vi "Scan DQMH Modules.vi"(8 "error in":errorcluster) -> (0 "error out":errorcluster, 1 "Cloneable?":bool[](array[boolean]), 2 "Modules List":string[](array[string]), 3 "DQMH Modules":refnum<vi>[](array[refnum]))   [LabVIEW 2020, in "DQMH_API.lvlib"]
doc: "Gets the Singleton and Cloneable references and creates a list of each type of DQMH Modules"
uses:
  DQMH_API.lvlib
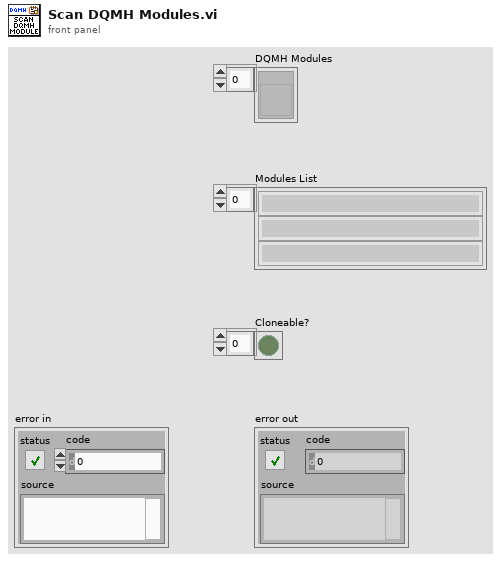
[diagram p1: front panel]
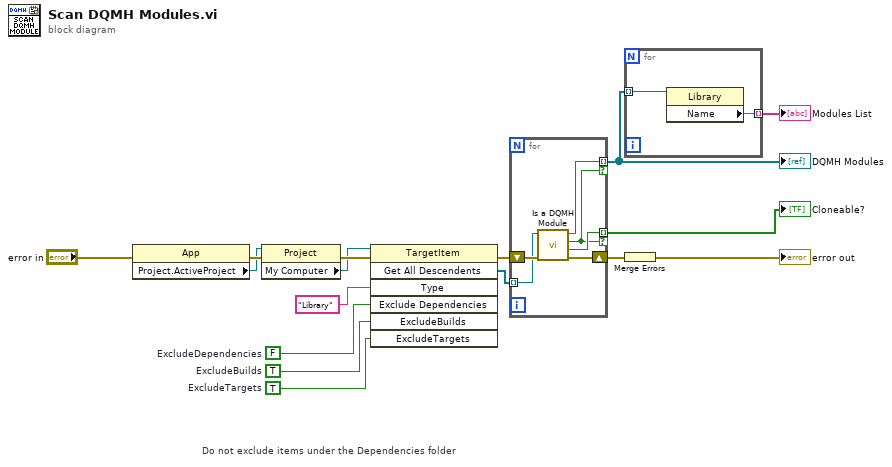
[diagram p0: block diagram]
diagram:
  w5 = FALSE  # ExcludeDependencies
  w6 = TRUE  # ExcludeTargets
  w7 = TRUE  # ExcludeBuilds
  # "Do not exclude items under the Dependencies folder"
  n1 = property class="App"(error in="error in") -> (error out=w14:errorcluster, "Project.ActiveProject"=w9:refnum<vi>)  [unwired: 1 in, 1 out]
  n2 = property class="Project"(reference=w9, error in=w14) -> (error out=w15:errorcluster, "My Computer"=w8:refnum<vi>)  [unwired: 1 out]
  n3 = invoke class="TargetItem" method="Get All Descendents"(reference=w8, error in=w15, "Type"="Library", "Exclude Dependencies"=w5, "ExcludeBuilds"=w7, "ExcludeTargets"=w6) -> (error out=w16:errorcluster, "All Descendents"=w4:refnum<vi>[])  [unwired: 1 in, 5 out]
  n4 = for {
    tunnel: w4 -> [w20] mode=indexing
    tunnel: [w19] -> w2 mode=indexing if=w17
    tunnel: [w18] -> w1 mode=indexing if=w17
    shift-right: [w21] -> w11
    shift-left: w16 -> [w22]
    n5 = call "Is a DQMH Module.vi"("error in"=w22, "Library"=w20) -> ("error out"=w21:errorcluster, "Cloneable?"=w18:bool, "Is DQMH?"=w17:bool, "Library Refnum"=w19:refnum<vi>)  [unwired: 6 in]
  }
  "DQMH Modules" <- w2
  "Cloneable?" <- w1
  n6 = for {
    tunnel: [w24] -> w10 mode=indexing
    tunnel: w2 -> [w23] mode=indexing
    n7 = property class="Library"(reference=w23) -> ("Name"=w24:string)  [unwired: 1 in, 2 out]
  }
  "Modules List" <- w10
  n8 = Merge Errors(w11) -> (→"error out":errorcluster)
